vi "Lectura de datos LVM POR BLOQUE.vi"() -> ()   [LabVIEW 2020]
panel:
  in  "stop":bool
  out "Waveform Graph":dynamicdata(graph)
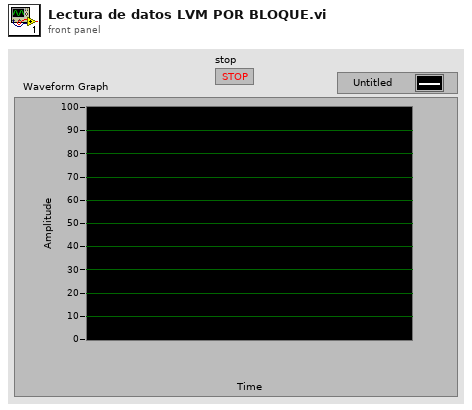
[diagram p1: front panel]
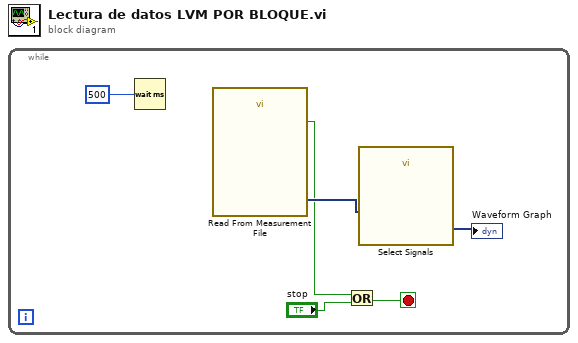
[diagram p0: block diagram]
diagram:
  n1 = while {
    stop <- w6 stop-if-true
    n2 = Wait (ms)(milliseconds to wait=u32 500) -> ()  [unwired: 1 out]
    n3 = call "Read From Measurement File"() -> ("Signals"=w3:dynamicdata, "EOF?"=w1:bool)  [unwired: 6 in, 4 out]
    n4 = Or(x=w1, y="stop") -> (x .or. y?=w6:bool)
    n5 = call "Select Signals"("Signals"=w3) -> ("Signal Out"=→"Waveform Graph":dynamicdata)  [unwired: 9 in, 1 out]
  }
